vi "Ping.vi"(11 "address":string="192.168.4.84") -> (3 "disconnected?":bool)   [LabVIEW 2025]
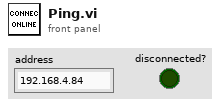
[diagram p1: front panel]
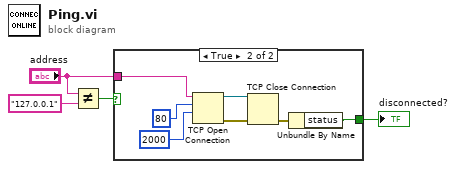
[diagram p0: block diagram]
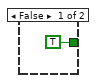
[diagram p2: hidden frame]
diagram:
  n1 = Not Equal?(x="address", y="127.0.0.1") -> (x != y?=w1:bool)
  n2 = case shown="True" w1 {
    tunnel: [TRUE ("status") w7] -> w4
    tunnel: "address" -> [_ w6]
    frame False {
    }
    frame True {
      n3 = TCP Open Connection(address=w6, remote port or service name=u16 80, timeout ms (60000)=2000) -> (connection ID=w11:refnum<k5>, error out=w12:errorcluster)  [unwired: 2 in]
      n4 = TCP Close Connection(connection ID=w11, error in (no error)=w12) -> (error out=w8:errorcluster)  [unwired: 1 in, 1 out]
      n5 = Unbundle By Name(w8) -> ("status"=w7:bool)
    }
  }
  "disconnected?" <- w4
